vi "Write VI name.vi"(5 "VI name":string, 9 "SubVI in":refnum<class "SubVI.lvclass">) -> (3 "SubVI out":refnum<class "SubVI.lvclass">)   [LabVIEW 2014]
uses:
  SubVI.lvclass
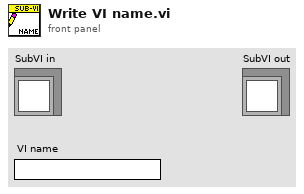
[diagram p1: front panel]
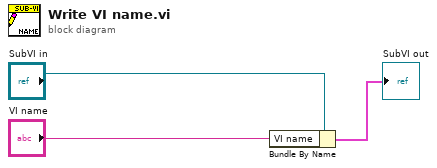
[diagram p0: block diagram]
diagram:
  n1 = Bundle By Name(cluster="SubVI in", "VI name"="VI name") -> (→"SubVI out":cluster{})
